vi "DriversStationData.vi"() -> ()   [LabVIEW 2018]
uses:
  Implements/Arm/TypeDefs/ArmAbsolutePosition.ctl
  General/MotionProfiling/TypeDefs/MPSendState.ctl
  Implements/Arm/TypeDefs/ArmHomingState.ctl
  Implements/Arm/TypeDefs/ArmTargetPosition.ctl
  General/MotionProfiling/TypeDefs/MotionProfileControlState.ctl
  Implements/Climber/TypeDefs/ClimberMode.ctl
  Implements/Climber/TypeDefs/ClimberHomingState.ctl
  Implements/Climber/TypeDefs/ClimberStates.ctl
panel:
  out "Arm Recovery Status":bool
  out "Arm Shoulder Failure Count":i16
  out "Arm Extension Failure Count":u16
  out "Arm Wrist Failure Count":u16
  in  "AutoClimberState":T1
  in  "Climber Home State":T2
  in  "ClimberMode":T3
  in  "Arm Mode":T4
  in  "Current Arm Position":T5
  in  "Armed Arm Position":T5
  in  "Arm Homing State":T6
  in  "Arm MP Send State":T7
  in  "Arm Position":T8
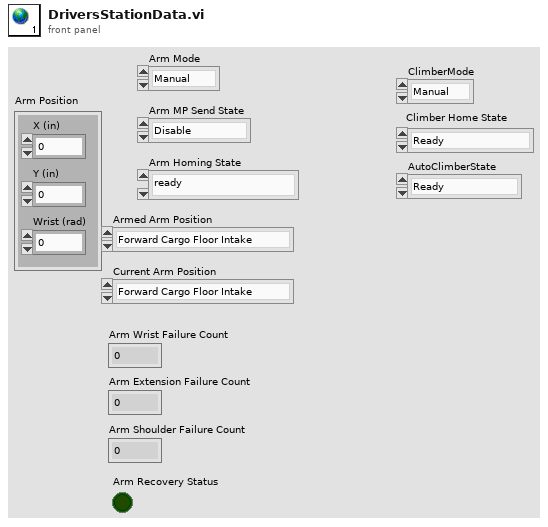
[diagram p1: front panel]
types:
  T1 = typedef "ClimberStates.ctl" = enum16{"Ready ", "Lift Bot ", "Raised Drive", "Raise Front Sticks ", "Raise Back Sticks ", "Park ", "Cancel"}
  T2 = typedef "ClimberHomingState.ctl" = enum16{"Ready", "Homing In progress", "Homing Failure", "Homing Success "}
  T3 = typedef "ClimberMode.ctl" = enum16{"Manual", "Auto", "Homing"}
  T4 = typedef "MotionProfileControlState.ctl" = enum16{"Manual", "Auto_Idle", "Auto_Run"}
  T5 = typedef "ArmTargetPosition.ctl" = enum16{"Forward Cargo Floor Intake", "Forward Cargo Feeder Station", "Forward Cargo Low", "Forward Cargo Middle", "Forward Cargo High", "Forward Cargo CargoShip", "Forward Hatch Floor Intake", "Forward Hatch Feeder Station", "Forward Hatch Low", "Forward Hatch Middle", "Forward Hatch High", "Forward Hatch CargoShip", "Reverse Cargo Floor Intake", "Reverse Cargo Feeder Station", "Reverse Cargo Low", "Reverse Cargo Middle", "Reverse Cargo High", "Reverse Cargo CargoShip", "Reverse Hatch Floor Intake", "Reverse Hatch Feeder Station", "Reverse Hatch Low", "Reverse Hatch Middle", "Reverse Hatch High", "Reverse Hatch CargoShip", "Hold"}
  T6 = typedef "ArmHomingState.ctl" = enum16{"ready", "homing in progress", "homing complete ", "homing failed"}
  T7 = typedef "MPSendState.ctl" = enum16{"Disable", "Commit Points", "Enable", "Done", "Failed"}
  T8 = typedef "ArmAbsolutePosition.ctl" = cluster{"X (in)":dbl, "Y (in)":dbl, "Wrist (rad)":dbl}
diagram:
